vi "Test_for_RapidScan.vi"() -> ()   [LabVIEW 2022 SP3]
uses:
  <vilib>/Motion/FlexMotion/CustomControls/CustomControls.llb/AxisOrVectorSpace To Control.flx
panel:
  out "End Position":i32
  in  "Total steps":i32
  in  "# frames / s":i32
  in  "Step interval":i32=1
  in  "start":bool
  in  "stop":bool
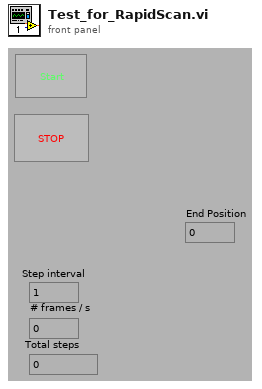
[diagram p1: front panel]
types:
  T1 = typedef "AxisOrVectorSpace To Control.flx" = u16
  T2 = typedef "Bd Id Out" = u8
  T3 = typedef "Resource Out (Enum).flx" = u16
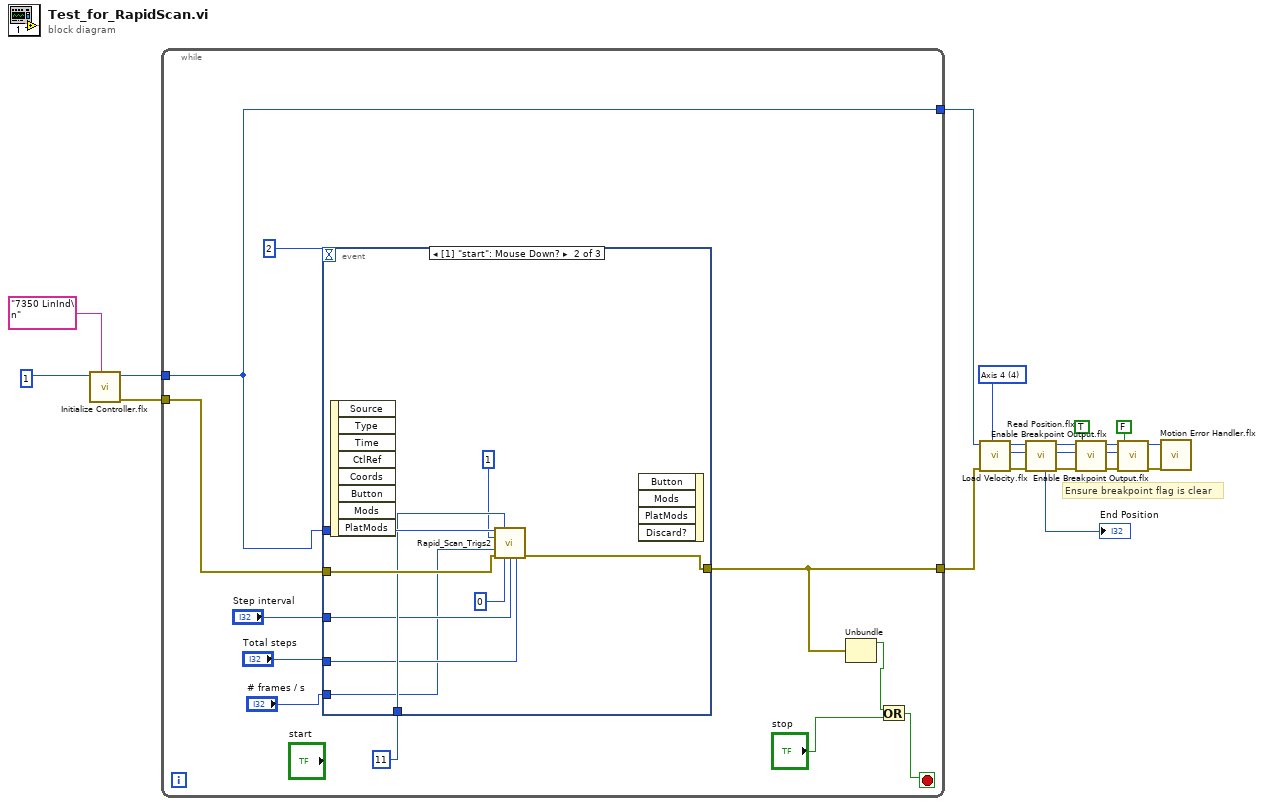
[diagram p0: block diagram]
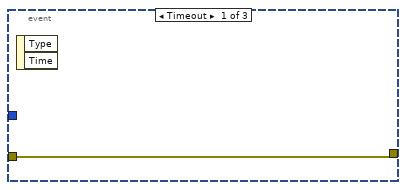
[diagram p2: hidden frame]
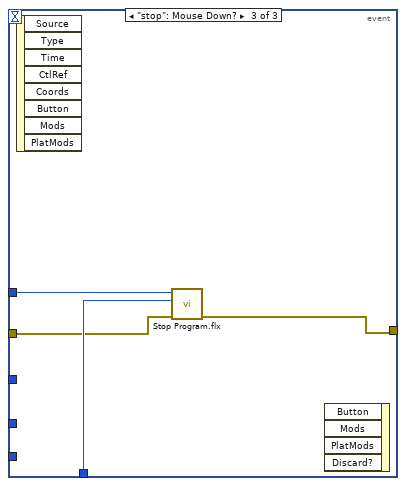
[diagram p3: hidden frame]
diagram:
  w1 = T1 4 items=["Axis 1"=1, "Axis 2"=2, "Axis 3"=3, "Axis 4"=4, "Axis 5"=5, "Axis 6"=6, "Axis 7"=7, "Axis 8"=8, "Vector Space 1"=17, "Vector Space 2"=18, "Vector Space 3"=19, "Vector Space 4"=20] ("Axis or Vector Space")
  # "Ensure breakpoint flag is clear"
  n1 = call <vilib>:"Initialize Controller.flx"("Settings Name"="7350 LinInd\n", "Board ID"=1) -> ("error out"=w3:errorcluster, "Bd ID Out"=w4:T2)  [unwired: 6 in]
  n2 = while {
    tunnel: [w29] -> w7
    tunnel: [w25] -> w6
    tunnel: w4 -> [w25]
    tunnel: w3 -> [w24]
    stop <- w28 stop-if-true
    n3 = event shown="[1] \"start\": Mouse Down?" {
      selector: _ -> [_ _ _]
      dyn-events: _ -> [_ _ _]
      timeout: 2 -> [_ _ _]
      tunnel: [w33 w39 w44] -> w29
      tunnel: w25 -> [_ w42 w46]
      tunnel: "Total steps" -> [_ w38 _]
      tunnel: "# frames / s" -> [_ w36 _]
      tunnel: 11 -> [_ w40 w45]
      tunnel: w24 -> [w33 w41 w43]
      tunnel: "Step interval" -> [_ w37 _]
      event Timeout {
        n4 = event-data() -> ()  [unwired: 1 in, 2 out]
      }
      event "start": Mouse Down? {
        n5 = event-data() -> ()  [unwired: 1 in, 8 out]
        n6 = call "Rapid_Scan_Trigs2.vi"("Board ID"=w42, "Program (1)"=w40, "Scan Axis"=1, "# frames/ s"=w36, "error in (no error)"=w41, "overshoot"=0, "step interval"=w37, "Total Steps (one way)"=w38) -> ("error out"=w39:errorcluster)  [unwired: 4 in, 3 out]
        n7 = event-data() -> ()  [unwired: 5 in, 1 out]
      }
      event "stop": Mouse Down? {
        n8 = event-data() -> ()  [unwired: 1 in, 8 out]
        n9 = call <vilib>:"Stop Program.flx"("error in (no error)"=w43, "Program (1)"=w45, "Board ID"=w46) -> ("error out"=w44:errorcluster)  [unwired: 3 in, 2 out]
        n10 = event-data() -> ()  [unwired: 5 in, 1 out]
      }
    }
    n11 = Unbundle(w29) -> ("status"=w26:bool)  [unwired: 2 out]
    n12 = Or(x=w26, y="stop") -> (x .or. y?=w28:bool)
  }
  n13 = call <vilib>:"Load Velocity.flx"("error in (no error)"=w7, "Axis or Vector Space"=w1, "Board ID"=w6) -> ("error out"=w20:errorcluster, "Resource Output"=w19:T3, "Bd ID Out"=w21:T2)  [unwired: 4 in]
  n14 = call <vilib>:"Read Position.flx"("error in (no error)"=w20, "Axis"=w19, "Board ID"=w21) -> ("error out"=w16:errorcluster, "Resource Output"=w15:T3, "Bd ID Out"=w17:T2, "Position"=→"End Position":i32)  [unwired: 3 in]
  n15 = call <vilib>:"Enable Breakpoint Output.flx"("Enable Breakpoint"=TRUE, "error in (no error)"=w16, "Axis or Encoder"=w15, "Board ID"=w17) -> ("error out"=w13:errorcluster, "Resource Output"=w10:T3, "Bd ID Out"=w14:T2)  [unwired: 3 in]
  n16 = call <vilib>:"Enable Breakpoint Output.flx"("Enable Breakpoint"=FALSE, "error in (no error)"=w13, "Axis or Encoder"=w10, "Board ID"=w14) -> ("error out"=w11:errorcluster, "Bd ID Out"=w12:T2)  [unwired: 3 in, 1 out]
  n17 = call <vilib>:"Motion Error Handler.flx"("Board ID"=w12, "error in (no error)"=w11) -> ()  [unwired: 9 in, 5 out]
